vi "Write Events.vi"(8 "error in (no error)":errorcluster, 10 "Events":T1, 11 "Panel Event Msg in":refnum<class "Panel Event Msg.lvclass">) -> (0 "error out":errorcluster, 3 "Panel Event Msg out":refnum<class "Panel Event Msg.lvclass">)   [LabVIEW 2021, in "Panel Event.lvlib" / "Panel Event Msg.lvclass"]
uses:
  Panel Event Msg.lvclass
  Events.ctl
  Panel Event Msg.lvclass/Panel Event Msg.ctl
  Panel Event.lvlib
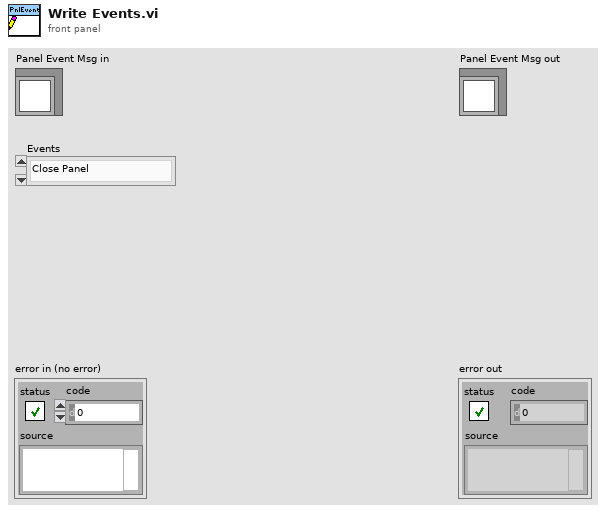
[diagram p1: front panel]
types:
  T1 = typedef "Panel Event.lvlib/Events.ctl" = enum16{"Close Panel", "Show Panel", "Hide Panel"}
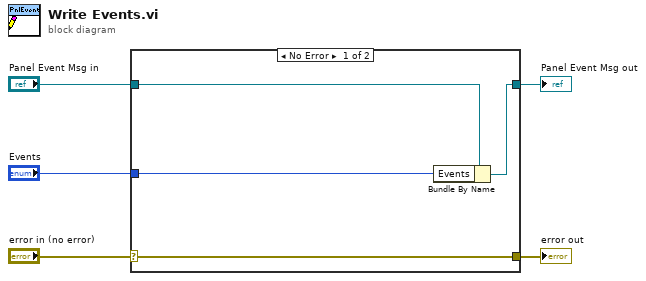
[diagram p0: block diagram]
diagram:
  n1 = case shown="No Error" "error in (no error)" {
    selector: "error in (no error)" -> [w9 w10]
    tunnel: [w9 w10] -> w4
    tunnel: [w7 w11] -> w2
    tunnel: "Panel Event Msg in" -> [w8 w11]
    tunnel: "Events" -> [w6 _]
    frame No Error {
      n2 = Bundle By Name(cluster=w8, "Events"=w6) -> (w7:refnum<class "Panel Event Msg.lvclass">)
    }
    frame Error {
    }
  }
  "error out" <- w4
  "Panel Event Msg out" <- w2
